vi "Delete all cursors.vi"(0 "Display State In":T1, 9 "Container State":T2, 11 "error in (no error)":errorcluster) -> (4 "Display State Out":T1, 15 "error out":errorcluster)   [LabVIEW 2014, in "Graph with cursors XControl.xctl"]
uses:
  Graph with cursors XControl.xctl
  <vilib>/_xctls/Container State.ctl
  Graph with cursors State.ctl
  <vilib>/Utility/miscctls.llb/LVCursorListTypeDef.ctl
  <vilib>/_xctls/XControlSupport.lvlib
panel:
  # "Add Controls & Indicators that form the parameters of the method here. Hook them to the connector pane. Do not delete the controls & indicators that are already hooked to the connector pane.\n \nTo setup the parameters  for this method, right click on this item in the Project Tree & select \"Configure Method...\"."
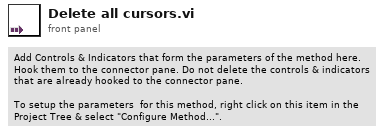
[diagram p1: front panel]
types:
  T1 = typedef "Graph with cursors XControl.xctl/Graph with cursors State.ctl" = cluster{"Cursor names":string[], "Cursor positions":dbl[], "Cursor pairs":i32, "Graph":refnum<vi>, "Prefix":string, "Base path":path}
  T2 = typedef "XControlSupport.lvlib/Container State.ctl" = cluster{"Indicator?":bool, "Run Mode?":bool, " Refnum":refnum<vi>}
  T3 = typedef "LVCursorListTypeDef.ctl" = cluster{"Name":string, "Color":u32, "Style":u8, "Point Style":u8, "Name Visible":bool, "Allow Drag":bool, "Cursor Mode":u32, "Plot":i32, "Index":i32, "Position":cluster{"X":dbl, "Y":dbl}, "X Scale":u32, "Y Scale":u32, "Watch Plots":i32[], "Watch All Plots":bool, "Plot Area":i32, "Label Offset":cluster{"X":dbl, "Y":dbl}}[]
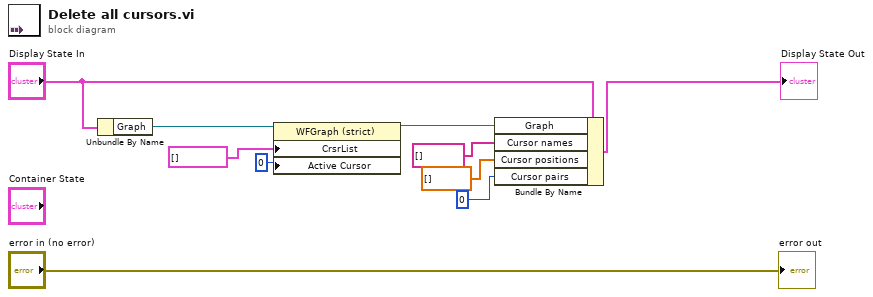
[diagram p0: block diagram]
diagram:
  n1 = Unbundle By Name("Display State In") -> ("Graph"=w9:refnum<vi>)
  n2 = property class="WFGraph (strict)"(reference=w9, "CrsrList"=T3 [] ("Cursor List"), "Active Cursor"=u32 0) -> (reference out=w5:refnum<vi>)  [unwired: 1 in, 1 out]
  n3 = Bundle By Name(cluster="Display State In", "Graph"=w5, "Cursor names"=string[] [], "Cursor positions"=dbl[] [], "Cursor pairs"=0) -> (→"Display State Out":T1)
  "error out" <- "error in (no error)"
